vi "Main XY controller.vi"() -> ()   [LabVIEW 2015]
uses:
  <vilib>/Utility/error.llb/DialogType.ctl
  <vilib>/DAQmx/read.llb/DAQmx Read (Counter DBL 1Chan 1Samp).vi
  <vilib>/DAQmx/read.llb/DAQmx Read (Digital Bool 1Line 1Point).vi
  <vilib>/DAQmx/write.llb/DAQmx Write (Analog DBL 1Chan 1Samp).vi
  <vilib>/DAQmx/create/channels.llb/DAQmx Create Channel (DI-Digital Input).vi
  <vilib>/DAQmx/create/channels.llb/DAQmx Create Channel (CI-Count Edges).vi
  <vilib>/DAQmx/create/channels.llb/DAQmx Create Channel (AO-Voltage-Basic).vi
  <vilib>/addons/control/pid/pid.llb/PID (DBL).vi
  <vilib>/imath/engines/lvmath2/RunTimeEngine/RangeToken/NIMS_Range.vi
  <instcachedir>/0/NIMS_Range_D919CC09935940E88F755EC1C6F49AC1.lvgen/NIMS_Range_D919CC09935940E88F755EC1C6F49AC1_000.vi
  <vilib>/imathl/engines/lvmath/Functions/Error Handling/Create Error.vi
  <vilib>/imath/engines/lvmath2/RunTimeEngine/IndexRead/NIMS V(S).vi
  <instcachedir>/0/NIMS V(S)_0488751826AF41519A22953C041130DC.lvgen/NIMS V(S)_0488751826AF41519A22953C041130DC_002.vi
  <vilib>/imath/engines/lvmath2/RunTimeEngine/RowToken/NIMS_RowToken_CV_CV.vi
  <instcachedir>/0/NIMS_RowToken_CV_CV_D10E7D21517B46419B9BC15369A9C889.lvgen/NIMS_RowToken_CV_CV_D10E7D21517B46419B9BC15369A9C889_000.vi
  <vilib>/imath/engines/lvmath2/RunTimeEngine/ErrorHandling/NIMS_Create Error From Enums.vi
  <vilib>/imath/engines/lvmath2/RunTimeSupport/NIMS_Error if Not Equal.vi
  <instcachedir>/0/NIMS_Error if Not Equal_7F0D61CE56BF44979916ECA34C78675F.lvgen/NIMS_Error if Not Equal_7F0D61CE56BF44979916ECA34C78675F_001.vi
  <vilib>/imath/engines/lvmath2/RunTimeEngine/IndexRead/NIMS M(V,S).vi
  <instcachedir>/0/NIMS M(V,S)_4A7282EC9BD94252BB5D44AC841A97D6.lvgen/NIMS M(V,S)_4A7282EC9BD94252BB5D44AC841A97D6_000.vi
  <vilib>/imath/engines/lvmath2/RunTimeEngine/IndexReplace/NIMS V(V)=V.vi
  <instcachedir>/0/NIMS V(V)=V_422D7BAD0B0F4E4DA085EB3347135799.lvgen/NIMS V(V)=V_422D7BAD0B0F4E4DA085EB3347135799_000.vi
  <vilib>/imath/engines/lvmath2/RunTimeEngine/IndexRead/NIMS M($,S).vi
  <instcachedir>/0/NIMS M($,S)_3E5749BBB62E49528D4765A77F1F6D98.lvgen/NIMS M($,S)_3E5749BBB62E49528D4765A77F1F6D98_000.vi
  <vilib>/imath/engines/lvmath2/RunTimeEngine/NodeEndStatement/NIMS_NodeEndStatement_Output.vi
  <instcachedir>/0/NIMS_NodeEndStatement_Output_53EC0D466D134D7ABD903AC30B43404B.lvgen/NIMS_NodeEndStatement_Output_53EC0D466D134D7ABD903AC30B43404B_005.vi
  <vilib>/imath/engines/lvmath2/RunTimeEngine/ErrorHandling/NIMS_Finalize Error.vi
  <instcachedir>/0/NIMS_Error if Not Equal_7F0D61CE56BF44979916ECA34C78675F.lvgen/NIMS_Error if Not Equal_7F0D61CE56BF44979916ECA34C78675F_000.vi
  <instcachedir>/0/NIMS V(S)_0488751826AF41519A22953C041130DC.lvgen/NIMS V(S)_0488751826AF41519A22953C041130DC_000.vi
  <vilib>/imath/engines/lvmath2/RunTimeEngine/VariableToken/NIMS_VariableToken_CondDefined.vi
  <instcachedir>/0/NIMS_VariableToken_CondDefined_FE30D0A1BFB24F098D41DEBABFE96BE1.lvgen/NIMS_VariableToken_CondDefined_FE30D0A1BFB24F098D41DEBABFE96BE1_004.vi
  <vilib>/imath/engines/lvmath/Functions/Error Handling/MergeErrorsWrapper.vi
  <instcachedir>/0/NIMS_NodeEndStatement_Output_53EC0D466D134D7ABD903AC30B43404B.lvgen/NIMS_NodeEndStatement_Output_53EC0D466D134D7ABD903AC30B43404B_001.vi
  <vilib>/DAQmx/miscellaneous.llb/DAQmx Fill In Error Info.vi
  <vilib>/addons/control/pid/NI_PID_pid.lvlib
panel:
  out "EncoderB":dbl
  out "EncoderA":dbl
  out "StoredM2":dbl
  out "StoredM1":dbl
  out "M2":dbl format="%0.2f"
  out "M1":dbl format="%0.2f"
  out "X Response":cluster{"X Pos":dbl, "Height 2":dbl}(graph)
  in  "stop":bool
  out "X Pos":dbl
  out "Y Pos":dbl
  out "Motor 1 Voltage":dbl
  out "Motor 2 Voltage":dbl
  out "Position (mm)":cluster{"X":dbl[], "Y":dbl[]}[](graph)
  out "Left Limit LED":bool
  out "Right Limit LED":bool
  out "Bottom Limit LED":bool
  out "Top Limit LED":bool
  in  "Speed Polling Rate":dbl=0.1 caption="Time Target (s)"
  out "Motor 2 Speed":dbl(knob) scale=0.0..100.0
  out "Motor 1 Speed":dbl(knob) scale=0.0..100.0
  out "Y Response":cluster{"X Pos":dbl, "Height 2":dbl}(graph)
  out "Motor 1  Voltage":dbl(graph)
  out "Motor 2 Voltage":dbl(graph)
  in  "Motion Control":T1(tab)
  in  "Acceleration":dbl=0.1 step=0.01
  in  "DL":bool
  out "Speed":dbl
  in  "Up":bool
  in  "R":bool
  in  "L":bool
  in  "Down":bool
  in  "UR":bool
  in  "DR":bool
  in  "UL":bool
  in  "Motor Offset 1":dbl=1.0 step=0.01 format="%#_13g"
  in  "Motor Offset 2":dbl=0.96 step=0.01 format="%#_13g"
  in  "Initial Speed":dbl=5.0
  in  "Height 2":dbl
  in  "Width 2":dbl
  in  "Go to position 3":bool
  out "Drawing? 2":bool
  out "Change State Flag 2":i32
  in  "PID gains":T2={"proportional gain (Kc)"=10.0, "integral time (Ti, min)"=0.1, "derivative time (Td, min)"=0.0}
  in  "dt (s)":dbl=20.0 format="%#_13g"
  in  "Max Speed":dbl(knob) scale=0.0..10.0
  in  "Reset Button":bool caption="OK Button"
  in  "State":u32
  in  "Max Speed":dbl=7.5
  out "Drawing?":bool
  in  "Draw Circle":bool
  in  "Height":dbl=50.0
  in  "Width":dbl=20.0
  out "StartingX":dbl
  out "StartingY":dbl
  out "Y Motor Control":dbl
  out "X Motor Contorl":dbl
  in  "Allowable Error":dbl=1.0
  in  "Up Limit":tag="Dev5/port0/line0"
  in  "Bottom Limit":tag="Dev5/port0/line1"
  in  "Right Limit":tag="Dev5/port0/line2"
  in  "Left Limit":tag="Dev5/port0/line3"
  in  "Motor 1 Encoder":tag="Dev5/ctr0"
  in  "Motor 2 Encoder":tag="Dev5/ctr1"
  in  "Motor2":tag="Dev5/ao1"
  in  "Motor1":tag="Dev5/ao0"
  in  "Max Voltage":dbl
  in  "Reinitialize X & Y Pos":bool
  in  "Speed (Voltage)":dbl
  in  "Go to position 2":bool
  out "Boolean 2":bool
  in  "Desired Y":dbl
  in  "Desired X":dbl
  out "X Motor Contorl 2":dbl
  out "Y Motor Control 2":dbl
  in  "Generate coordinates":bool
  out "Drawing?":bool
  in  "draw circle":bool
  in  "Radius":dbl=50.0
  in  "Points":dbl=300.0 step=180.0
  in  "Max Speed":dbl=5.0
  in  "Allowable Error 2":dbl=0.45
  in  "Point":u32
  out "StoredM2 2":dbl
  out "StoredM1 2":dbl
  out "M2 2":dbl format="%0.2f"
  out "M1 2":dbl format="%0.2f"
  out "ypos":dbl[](array[numeric])
  out "xpos":dbl[](array[numeric])
  out "Y Motor Control 4":dbl
  out "X Motor Contorl 4":dbl
  out "Storage 2":dbl
  out "Storage":dbl
  out "Desired plot X":dbl
  out "Desired Y plot":dbl
  out "X Motor Contorl 3":dbl
  out "Y Motor Control 3":dbl
  # "Naseeb Khan - NKHA186"
  # "XY Sliderail Controller"
  # "MECHENG 312"
  # "Daniel McGinn - DMCG924"
  # "All units in mm unless otherwise specifed"
  # "Limit Switches"
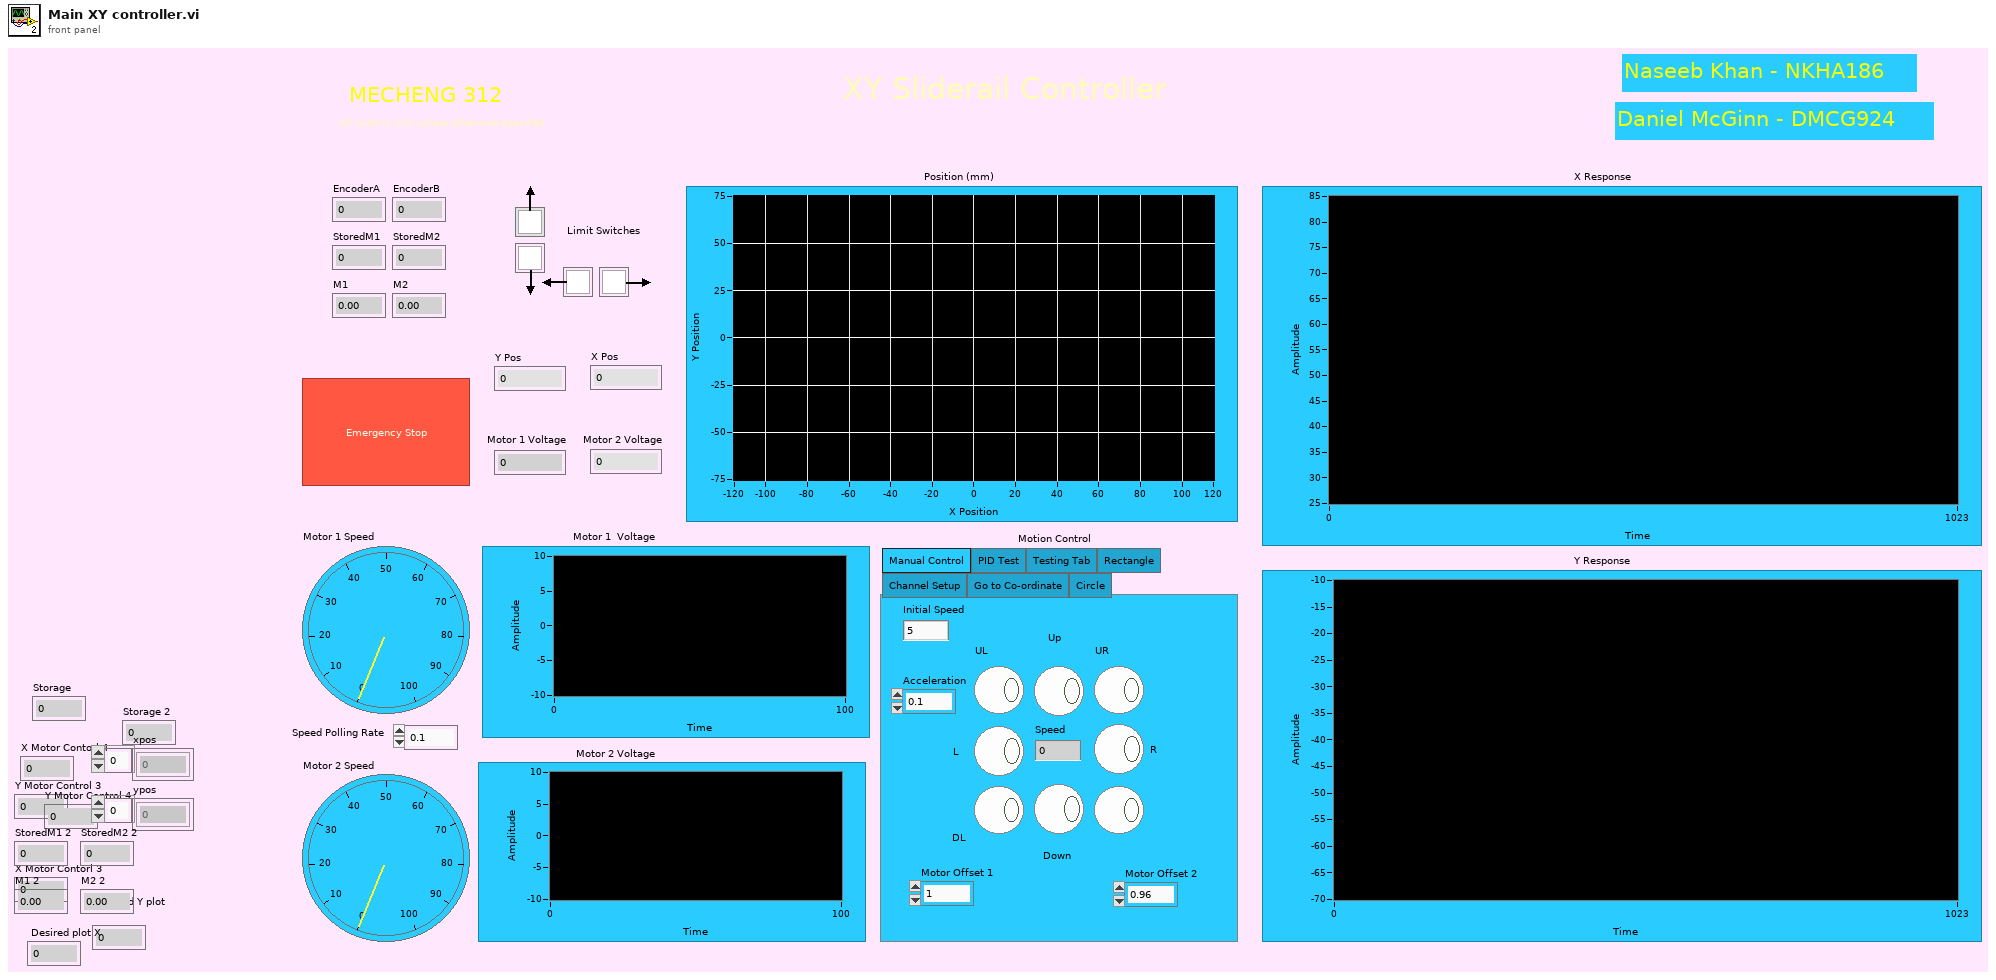
[diagram p1: front panel]
types:
  T1 = enum32{"Manual Control", "PID Test", "Testing Tab", "Rectangle", "Channel Setup", "Go to Co-ordinate", "Circle"}
  T2 = cluster{"proportional gain (Kc)":dbl, "integral time (Ti, min)":dbl, "derivative time (Td, min)":dbl}
  T3 = typedef "DialogType.ctl" = u16
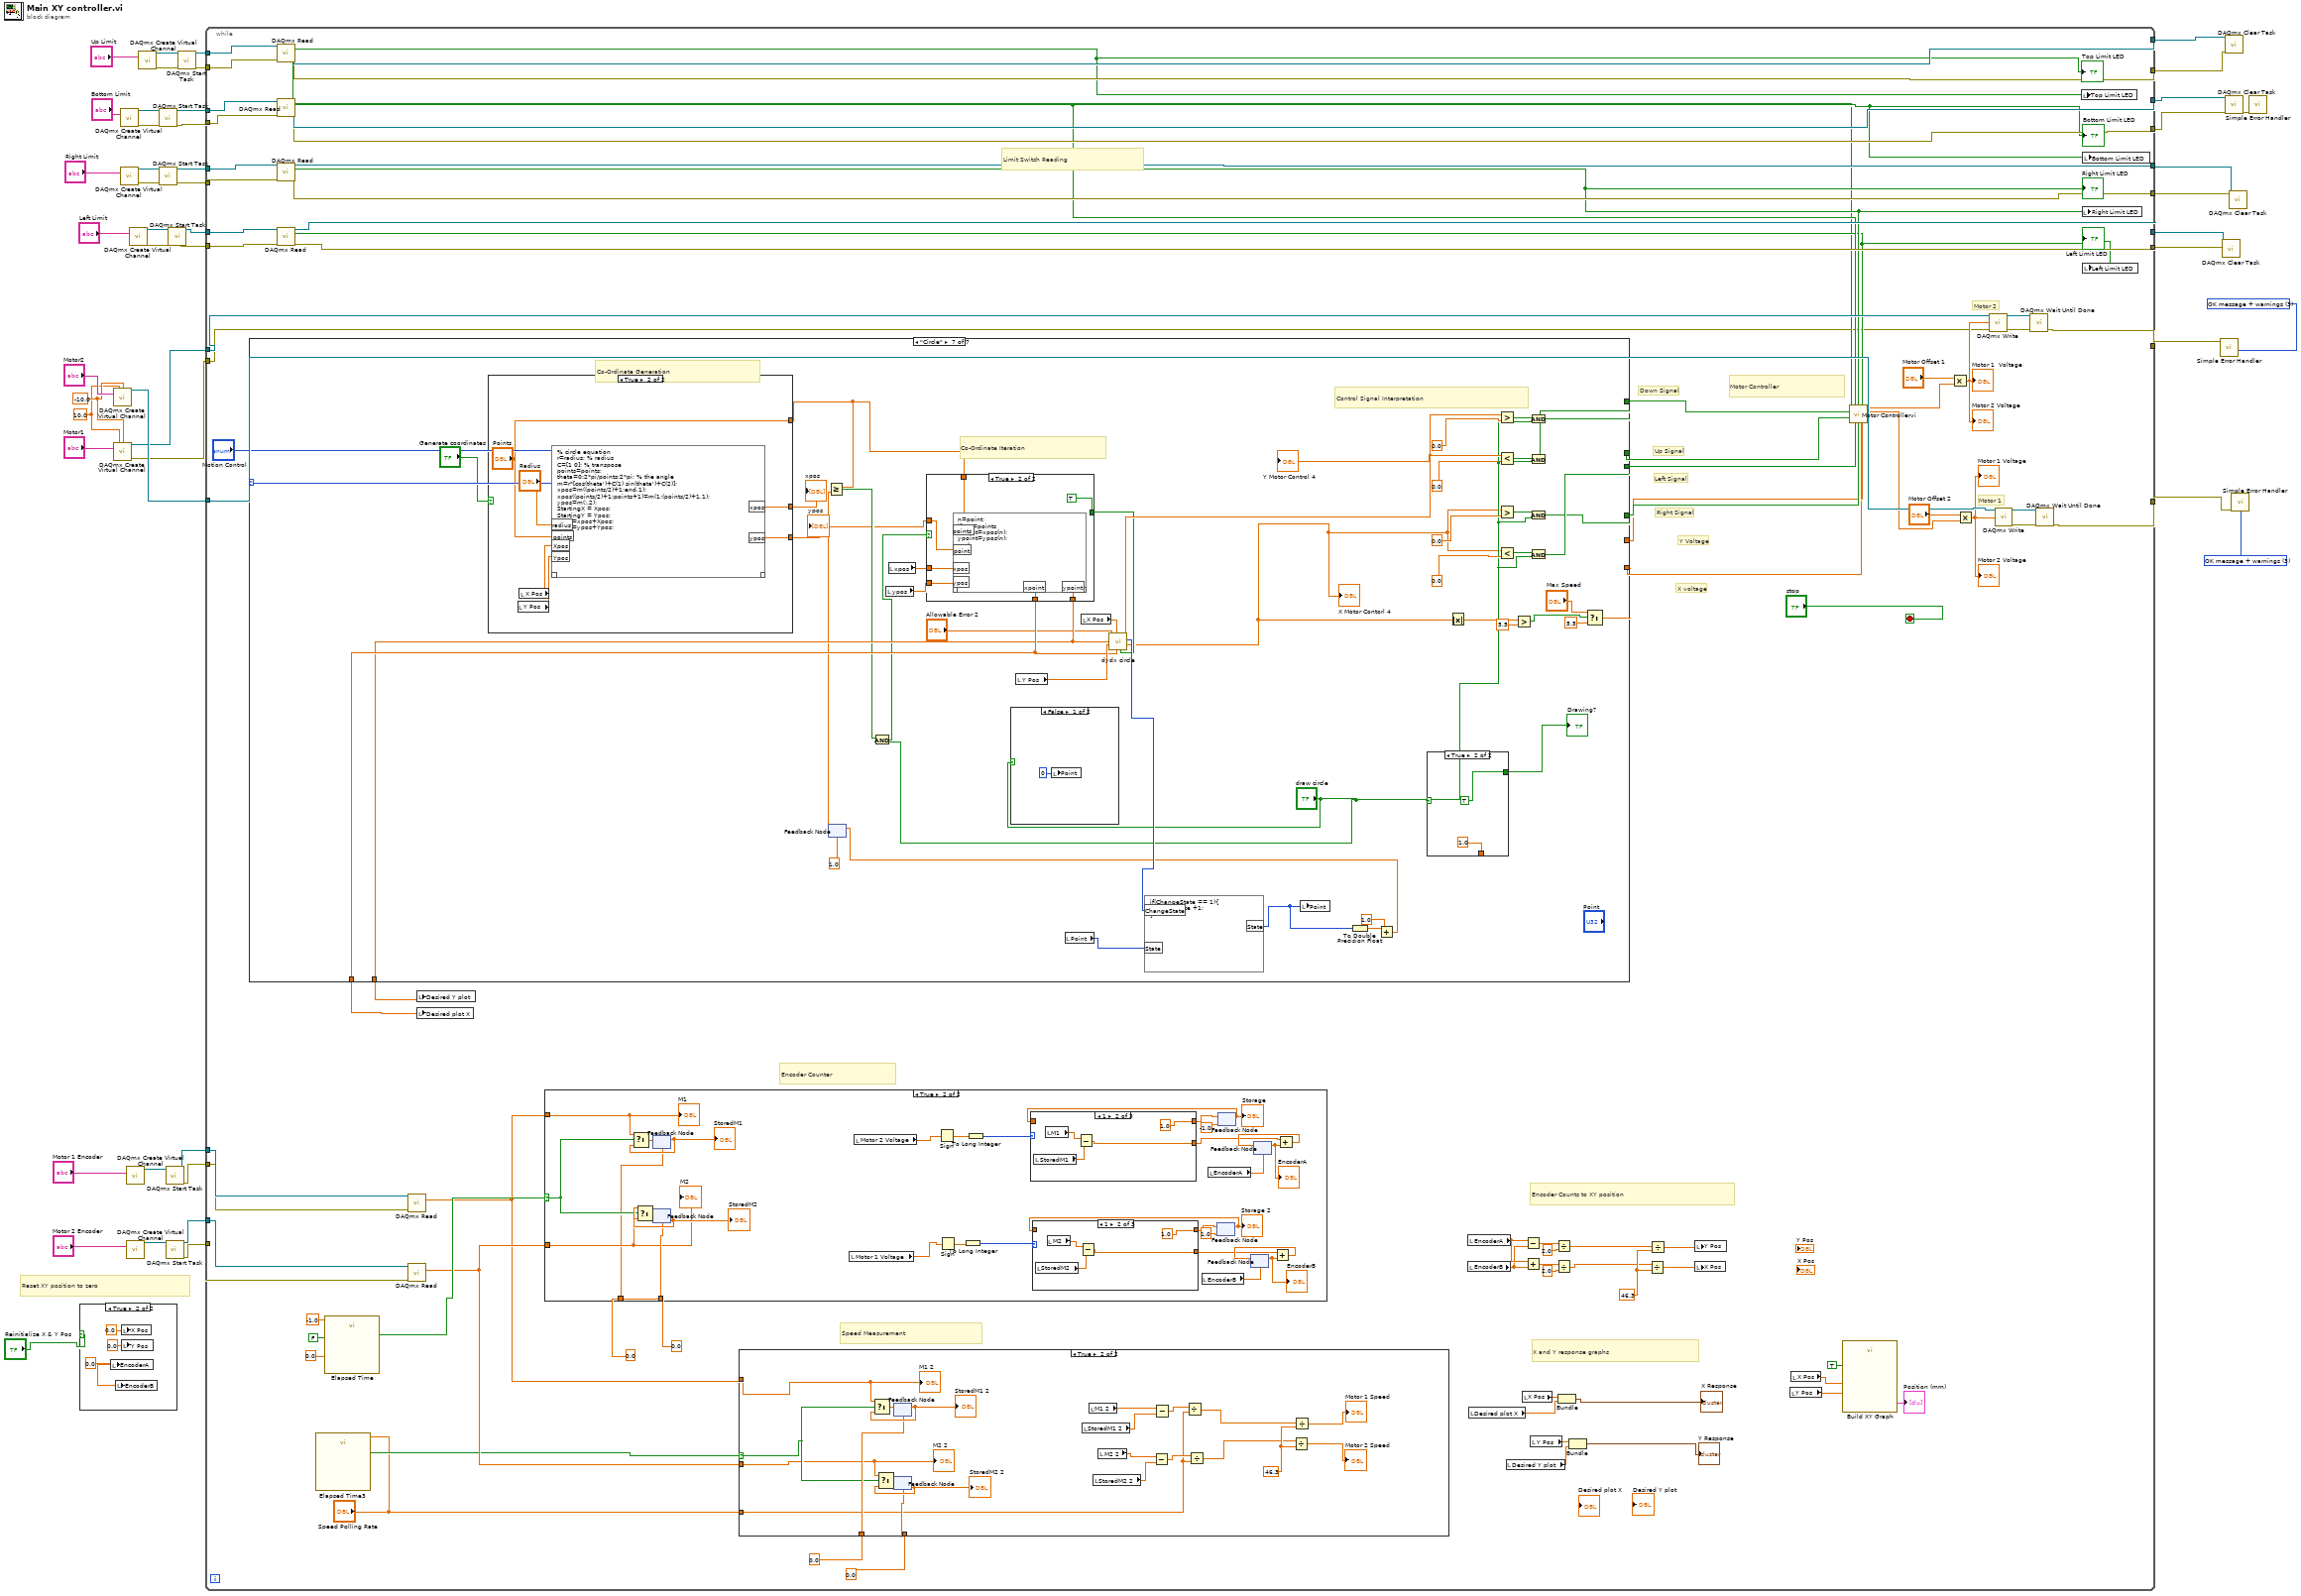
[diagram p0: block diagram]
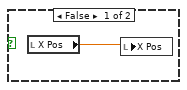
[diagram p2: hidden frame]
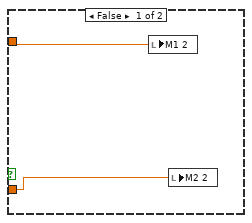
[diagram p3: hidden frame]
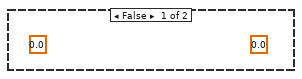
[diagram p4: hidden frame]
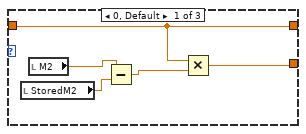
[diagram p5: hidden frame]
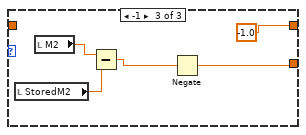
[diagram p6: hidden frame]
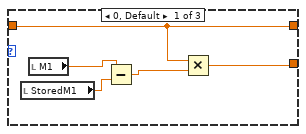
[diagram p7: hidden frame]
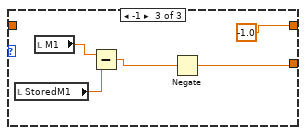
[diagram p8: hidden frame]
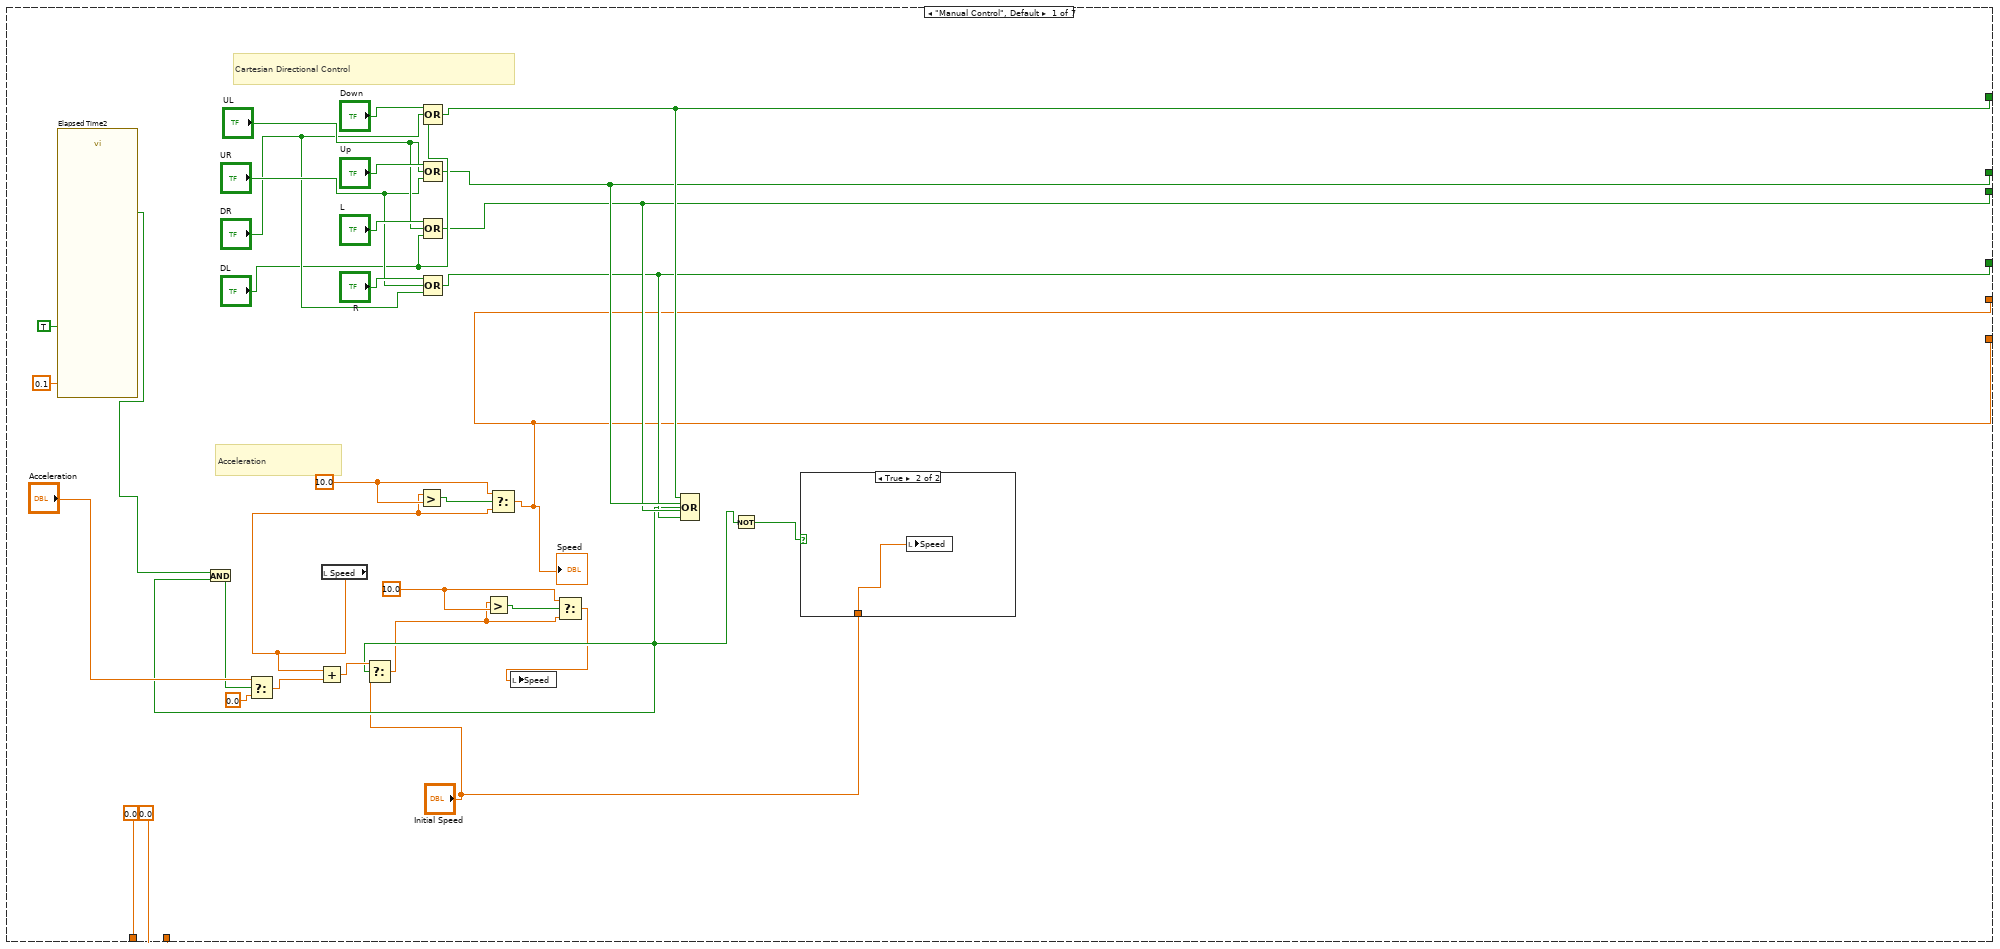
[diagram p9: hidden frame]
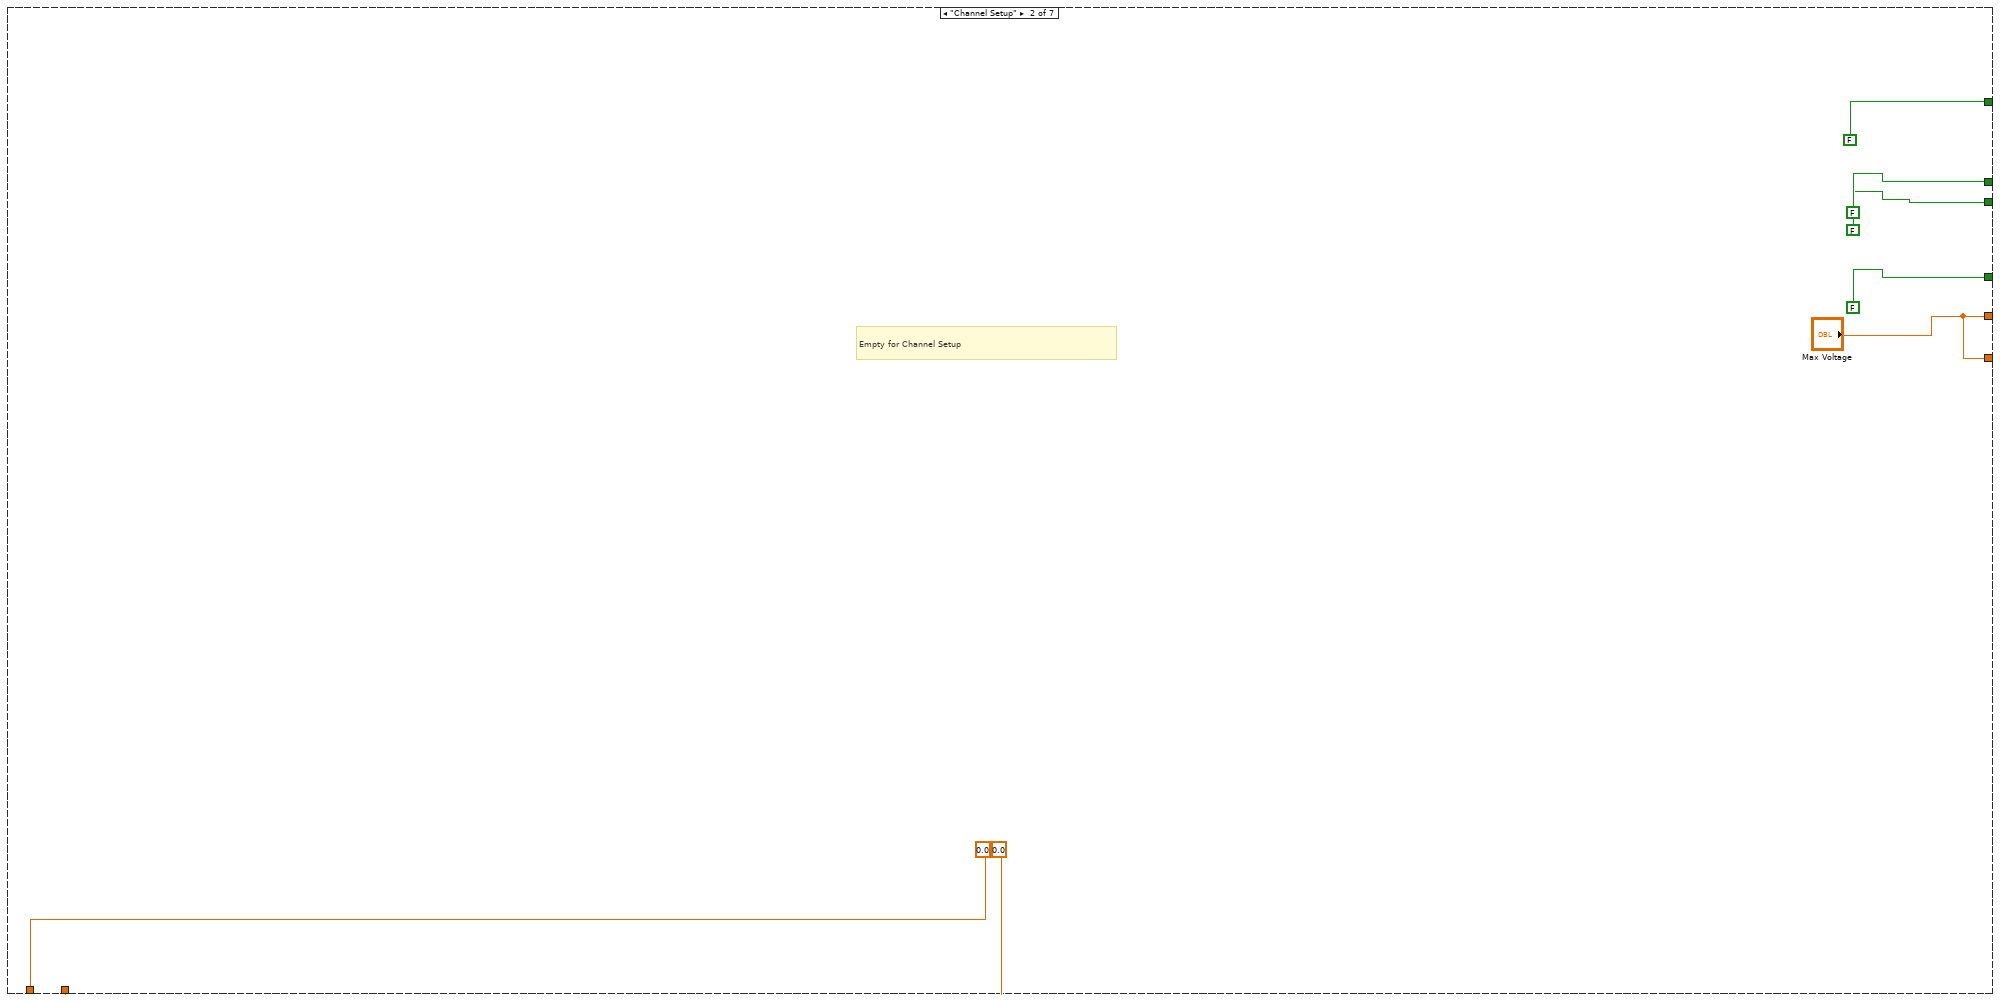
[diagram p11: hidden frame]
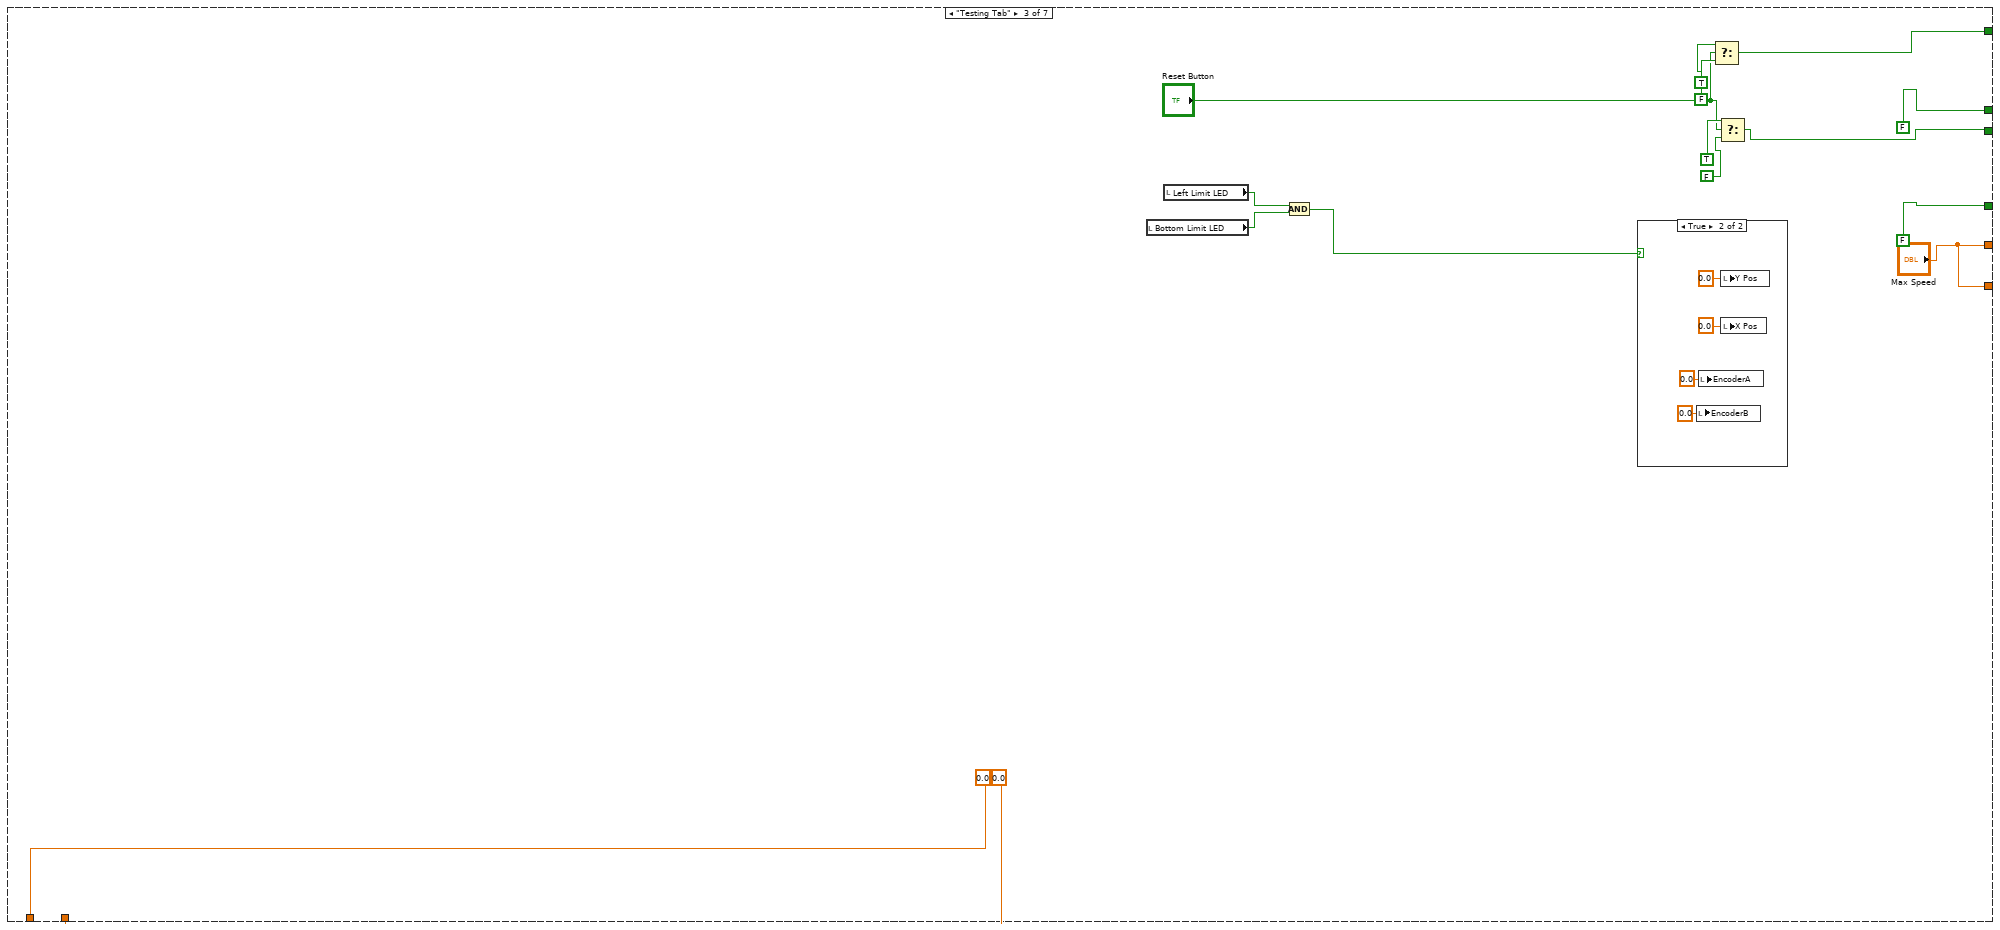
[diagram p12: hidden frame]
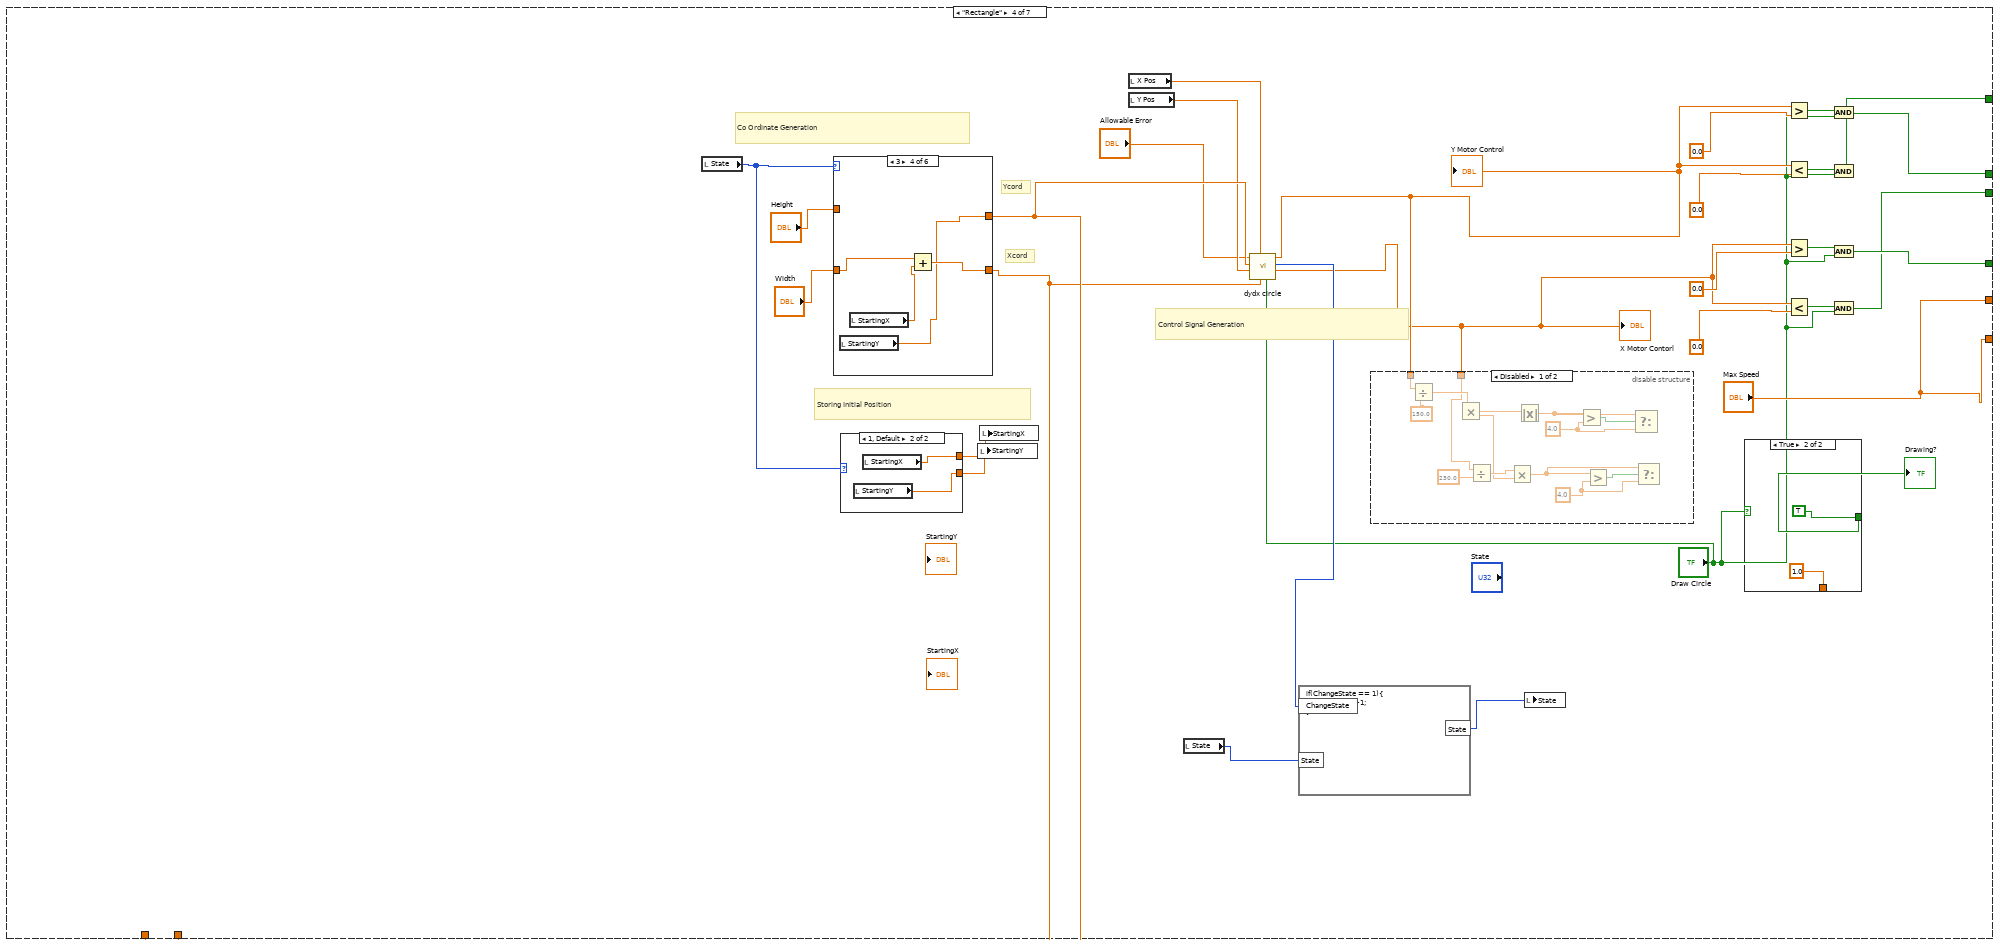
[diagram p14: hidden frame]
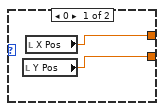
[diagram p16: hidden frame]
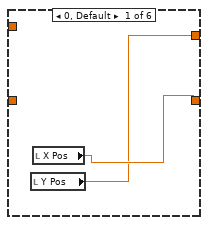
[diagram p17: hidden frame]
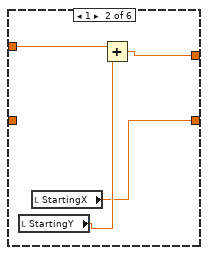
[diagram p18: hidden frame]
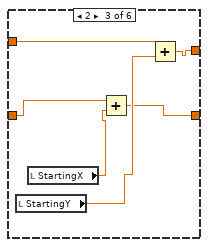
[diagram p19: hidden frame]
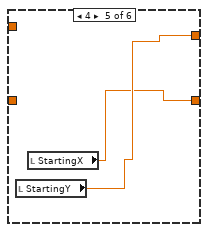
[diagram p20: hidden frame]
diagram:
  w10 = 10.0 ("Maximum Voltage")
  w11 = -10.0
  w44 = T3 3 items=["no dialog", "OK message", "continue or stop message", "OK message + warnings", "continue/stop + warnings"] ("type of dialog (OK msg:1)")
  w48 = T3 3 items=["no dialog", "OK message", "continue or stop message", "OK message + warnings", "continue/stop + warnings"] ("type of dialog (OK msg:1)")
  # "Reset XY position to zero"
  n1 = case shown="True" "Reinitialize X & Y Pos" {
    frame False {
      n2 = local read "X Pos"() -> (w50:dbl)
      n3 = local write "X Pos"(w50) -> ()
    }
    frame True {
      w51 = 0.0 ("NewEncoderPos")
      n4 = local write "EncoderA"(w51) -> ()
      n5 = local write "EncoderB"(w51) -> ()
      n6 = local write "X Pos"(0.0 ("X Pos")) -> ()
      n7 = local write "Y Pos"(0.0 ("Y Pos")) -> ()
    }
  }
  n8 = call-poly <vilib>:"DAQmx Create Virtual Channel.vi"("maximum value"=w10, "minimum value"=w11, "physical channels"="Motor2") -> ("task out"=w46:refnum<k21>)  [unwired: 11 in, 1 out]
  n9 = call-poly <vilib>:"DAQmx Create Virtual Channel.vi"("maximum value"=w10, "minimum value"=w11, "physical channels"="Motor1") -> ("task out"=w41:refnum<k21>, "error out"=w42:errorcluster)  [unwired: 11 in]
  n10 = call-poly <vilib>:"DAQmx Create Virtual Channel.vi"("lines"="Bottom Limit") -> ("task out"=w34:refnum<k21>, "error out"=w33:errorcluster)  [unwired: 13 in]
  n11 = call-poly <vilib>:"DAQmx Create Virtual Channel.vi"("lines"="Right Limit") -> ("task out"=w32:refnum<k21>, "error out"=w31:errorcluster)  [unwired: 13 in]
  n12 = call-poly <vilib>:"DAQmx Create Virtual Channel.vi"("counter"="Motor 1 Encoder") -> ("task out"=w1:refnum<k21>)  [unwired: 13 in, 1 out]
  n13 = call-poly <vilib>:"DAQmx Create Virtual Channel.vi"("counter"="Motor 2 Encoder") -> ("task out"=w7:refnum<k21>)  [unwired: 13 in, 1 out]
  n14 = call-poly <vilib>:"DAQmx Create Virtual Channel.vi"("lines"="Left Limit") -> ("task out"=w30:refnum<k21>, "error out"=w29:errorcluster)  [unwired: 13 in]
  n15 = call-poly <vilib>:"DAQmx Create Virtual Channel.vi"("lines"="Up Limit") -> ("task out"=w36:refnum<k21>, "error out"=w35:errorcluster)  [unwired: 13 in]
  n16 = call <vilib>:"DAQmx Start Task.vi"("task/channels in"=w34, "error in"=w33) -> ("task out"=w26:refnum<k21>, "error out"=w25:errorcluster)  [unwired: 12 in]
  n17 = call <vilib>:"DAQmx Start Task.vi"("task/channels in"=w32, "error in"=w31) -> ("task out"=w24:refnum<k21>, "error out"=w23:errorcluster)  [unwired: 12 in]
  n18 = call <vilib>:"DAQmx Start Task.vi"("task/channels in"=w1) -> ("task out"=w6:refnum<k21>, "error out"=w3:errorcluster)  [unwired: 13 in]
  n19 = call <vilib>:"DAQmx Start Task.vi"("task/channels in"=w7) -> ("task out"=w5:refnum<k21>, "error out"=w4:errorcluster)  [unwired: 13 in]
  n20 = call <vilib>:"DAQmx Start Task.vi"("task/channels in"=w30, "error in"=w29) -> ("task out"=w22:refnum<k21>, "error out"=w21:errorcluster)  [unwired: 12 in]
  n21 = call <vilib>:"DAQmx Start Task.vi"("task/channels in"=w36, "error in"=w35) -> ("task out"=w28:refnum<k21>, "error out"=w27:errorcluster)  [unwired: 12 in]
  n22 = while {
    tunnel: w46 -> [w133]
    tunnel: [w113] -> w45
    tunnel: [w132] -> w43
    tunnel: w42 -> [w62]
    tunnel: w41 -> [w131]
    tunnel: w28 -> [w130]
    tunnel: w27 -> [w129]
    tunnel: w26 -> [w128]
    tunnel: w25 -> [w127]
    tunnel: w24 -> [w126]
    tunnel: w23 -> [w125]
    tunnel: w22 -> [w124]
    tunnel: w21 -> [w123]
    tunnel: [w122] -> w20
    tunnel: [w121] -> w19
    tunnel: [w120] -> w18
    tunnel: [w119] -> w17
    tunnel: [w118] -> w16
    tunnel: [w117] -> w15
    tunnel: [w116] -> w14
    tunnel: [w115] -> w13
    tunnel: w6 -> [w87]
    tunnel: w5 -> [w86]
    tunnel: w4 -> [w55]
    tunnel: w3 -> [w85]
    stop <- "stop" stop-if-true
    w72 = 46.3
    # "Limit Switch Reading"
    # "Motor Controller"
    # "Speed Measurement"
    # "Encoder Counter"
    # "X and Y response graphs"
    # "Encoder Counts to XY position"
    # "Y Voltage"
    # "X voltage"
    # "Motor 1"
    # "Motor 2"
    # "Right Signal"
    # "Left Signal"
    # "Up Signal"
    # "Down Signal"
    n23 = case shown="\"Circle\"" "Motion Control" {
      tunnel: [w233 FALSE w264 w299 w377 w404 w438] -> w107
      tunnel: [w232 FALSE ("Up") FALSE ("Up") w300 w378 w405 w437] -> w106
      tunnel: [w230 FALSE ("Right\n 2") FALSE ("Right\n 2") w296 w374 w401 w435] -> w105
      tunnel: [w231 FALSE ("Left 2") w263 w295 w373 w400 w436] -> w99
      tunnel: [w220 "Max Voltage" "Max Speed" "Max Speed" w367 "Speed (Voltage)" w415] -> w97
      tunnel: [w220 "Max Voltage" "Max Speed" "Max Speed" w364 "Speed (Voltage)" w415] -> w96
      tunnel: [0.0 ("Desired Y") 0.0 ("Desired Y") 0.0 ("Desired Y") w284 "Width 2" "Desired X" w443] -> w89
      tunnel: [0.0 ("Desired X") 0.0 ("Desired X") 0.0 ("Desired X") w285 "Height 2" "Desired Y" w442] -> w88
      frame "Manual Control", Default {
        w218 = 10.0 ("y")
        w222 = 10.0 ("y")
        # "Cartesian Directional Control"
        # "Acceleration"
        n24 = call "Elapsed Time2"("Time Target (s)"=0.1, "Auto Reset"=TRUE) -> ("Time has Elapsed"=w229:bool)  [unwired: 10 in, 7 out]
        n25 = local read "Speed"() -> (w221:dbl)
        n26 = Greater?(x=w221, y=w222) -> (0:w223:bool)
        n27 = Compound Arithmetic op=OR("Down", "DR", "DL") -> (w233:bool)
        n28 = Compound Arithmetic op=OR("Up", "UL", "UR") -> (w232:bool)
        n29 = Compound Arithmetic op=OR("L", "UL", "DL") -> (w231:bool)
        n30 = Compound Arithmetic op=OR("R", "UR", "DR") -> (w230:bool)
        n31 = Select(t=w222, s=w223, f=w221) -> (s? t:f=w220:dbl)
        "Speed" <- w220
        n32 = Compound Arithmetic op=OR(w233, w232, w231, w230) -> (w225:bool)
        n33 = And(x=w229, y=w225) -> (x .and. y?=w228:bool)
        n34 = Select(t="Acceleration", s=w228, f=0.0) -> (s? t:f=w235:dbl)
        n35 = Add(x=w221, y=w235) -> (x+y=w226:dbl)
        n36 = Select(t=w226, s=w225, f="Initial Speed") -> (s? t:f=w217:dbl)
        n37 = Greater?(x=w217, y=w218) -> (0:w219:bool)
        n38 = Select(t=w218, s=w219, f=w217) -> (s? t:f=w216:dbl)
        n39 = local write "Speed"(w216) -> ()
        n40 = Not(x=w225) -> (.not. x?=w227:bool)
        n41 = case shown="True" w227 {
          tunnel: "Initial Speed" -> [_ w249]
          frame False {
          }
          frame True {
            n42 = local write "Speed"(w249) -> ()
          }
        }
      }
      frame "Channel Setup" {
        # "Empty for Channel Setup"
      }
      frame "Testing Tab" {
        n43 = local read "Bottom Limit LED"() -> (w261:bool)
        n44 = local read "Left Limit LED"() -> (w262:bool)
        n45 = And(x=w262, y=w261) -> (x .and. y?=w260:bool)
        n46 = case shown="True" w260 {
          frame False {
          }
          frame True {
            n47 = local write "EncoderB"(0.0 ("EncodB")) -> ()
            n48 = local write "EncoderA"(0.0 ("EncodA")) -> ()
            n49 = local write "Y Pos"(0.0 ("Y Pos")) -> ()
            n50 = local write "X Pos"(0.0 ("X Pos")) -> ()
          }
        }
        n51 = Select(t=TRUE, s="Reset Button", f=FALSE) -> (s? t:f=w264:bool)
        n52 = Select(t=TRUE, s="Reset Button", f=FALSE) -> (s? t:f=w263:bool)
      }
      frame "Rectangle" {
        # "Control Signal Generation"
        # "Storing Initial Position"
        # "Co Ordinate Generation"
        # "Ycord"
        # "Xcord"
        n53 = local read "State"() -> (w288:u32)
        n54 = case shown="3" w288 {
          tunnel: [w326 w327 w332 w338 w341 w343] -> w284
          tunnel: [w325 w328 w331 w337 w342 w344] -> w285
          tunnel: "Height" -> [_ w329 w336 _ _ _]
          tunnel: "Width" -> [_ _ w335 w340 _ _]
          frame 0, Default {
            n55 = local read "Y Pos"() -> (w325:dbl)
            n56 = local read "X Pos"() -> (w326:dbl)
          }
          frame 1 {
            n57 = local read "StartingY"() -> (w330:dbl)
            n58 = local read "StartingX"() -> (w327:dbl)
            n59 = Add(x=w329, y=w330) -> (x+y=w328:dbl)
          }
          frame 2 {
            n60 = local read "StartingY"() -> (w334:dbl)
            n61 = local read "StartingX"() -> (w333:dbl)
            n62 = Add(x=w335, y=w333) -> (x+y=w332:dbl)
            n63 = Add(x=w336, y=w334) -> (x+y=w331:dbl)
          }
          frame 3 {
            n64 = local read "StartingY"() -> (w337:dbl)
            n65 = local read "StartingX"() -> (w339:dbl)
            n66 = Add(x=w340, y=w339) -> (x+y=w338:dbl)
          }
          frame 4 {
            n67 = local read "StartingY"() -> (w342:dbl)
            n68 = local read "StartingX"() -> (w341:dbl)
          }
          frame 5 {
            n69 = local read "X Pos"() -> (w343:dbl)
            n70 = local read "Y Pos"() -> (w344:dbl)
            n71 = local write "State"(0) -> ()
          }
        }
        n72 = case shown="1, Default" w288 {
          tunnel: [w322 w324] -> w290
          tunnel: [w321 w323] -> w289
          frame 0 {
            n73 = local read "Y Pos"() -> (w321:dbl)
            n74 = local read "X Pos"() -> (w322:dbl)
          }
          frame 1, Default {
            n75 = local read "StartingY"() -> (w323:dbl)
            n76 = local read "StartingX"() -> (w324:dbl)
          }
        }
        n77 = local write "StartingY"(w289) -> ()
        n78 = local write "StartingX"(w290) -> ()
        n79 = local read "X Pos"() -> (w283:dbl)
        n80 = local read "Y Pos"() -> (w282:dbl)
        n81 = local read "State"() -> (w287:u32)
        n82 = call "dydx circle.vi"("count?"="Draw Circle", "Desired X in"=w284, "X Position"=w283, "Y Position"=w282, "Desired Y in"=w285, "Allowable Error 2"="Allowable Error") -> ("X Control"=w278:dbl, "ChangeState"=w280:i32, "Y Control"=w279:dbl)  [unwired: 3 in]
        "X Motor Contorl" <- w278
        "Y Motor Control" <- w279
        n83 = formula code="if(ChangeState == 1){\nState = State +1;\n}"("ChangeState"=w280, "State"=w287) -> ("State"=w286:u32)
        n84 = disable-structure shown="Disabled" {
          disable-tunnel: w279 -> [w319 _]
          disable-tunnel: w278 -> [w314 _]
          frame Disabled {
            w312 = 4.0 ("y")
            w310 = 4.0 ("y")
            n85 = Divide(x=w319, y=150.0) -> (x/y=w318:dbl)
            n86 = Multiply(x=w318) -> (y=w315:dbl, x*y=w308:dbl)
            n87 = Divide(x=w314, y=230.0) -> (x/y=w316:dbl)
            n88 = Multiply(x=w316, y=w315) -> (x*y=w306:dbl)
            n89 = Absolute Value(x=w308) -> (abs(x)=w307:dbl)
            n90 = Greater?(x=w307, y=w312) -> (0:w313:bool)
            n91 = Greater?(x=w306, y=w310) -> (0:w311:bool)
            n92 = Select(t=w307, s=w313, f=w312) -> ()  [unwired: 1 out]
            n93 = Select(t=w306, s=w311, f=w310) -> (s? t:f=w309:dbl)
          }
          frame Enabled {
          }
        }
        n94 = local write "State"(w286) -> ()
        n95 = case shown="True" "Draw Circle" {
          tunnel: [FALSE TRUE] -> w293
          tunnel: [0.0 1.0] -> _
          frame False {
          }
          frame True {
          }
        }
        "Drawing?" <- w293
        n96 = Greater?(x=w279, y=0.0) -> (0:w301:bool)
        n97 = Less?(x=w279, y=0.0) -> (x < y?=w298:bool)
        n98 = Greater?(x=w278, y=0.0) -> (0:w297:bool)
        n99 = Less?(x=w278, y=0.0) -> (x < y?=w294:bool)
        n100 = And(x=w301, y="Draw Circle") -> (x .and. y?=w300:bool)
        n101 = And(x=w298, y="Draw Circle") -> (x .and. y?=w299:bool)
        n102 = And(x=w297, y="Draw Circle") -> (x .and. y?=w296:bool)
        n103 = And(x=w294, y="Draw Circle") -> (x .and. y?=w295:bool)
      }
      frame "PID Test" {
        w365 = cluster{"output high":dbl, "output low":dbl} {"output high"=10.0, "output low"=-10.0} ("output range")
        # "Ignore"
        n104 = local read "X Pos"() -> (w363:dbl)
        n105 = local read "Y Pos"() -> (w368:dbl)
        n106 = formula code="float dY;\nfloat dX;\n\nint ChangeState = 0;\n\n dY = nextY - Yi;\n dX = nextX - Xi;\nint Xflag = 0;\nint Yflag = 0;\n\nif(( -0.5 > dY) || (dY > 0.5)){\nYcon = dY;\nYflag = 0;\n}\nelse{\nYcon = 0;\nYflag = 1;\n}\n\nif((-0.5 > dX) || (dX > 0.5)){\nXcon = dX;\nXflag = 0;\n}\nelse{\nXcon=0;\nXflag=1;\n}\n\nif((Xflag + Yflag )== 2){\nChangeState = 1;\n}"("Yi"=w368, "Xi"=w363, "nextY"="Height 2", "nextX"="Width 2") -> ("Ycon"=w359:dbl, "Xcon"=w357:dbl, "ChangeState"=→"Change State Flag 2":i32)
        n107 = call-poly <vilib>:"PID.vi"("output range"=w365, "dt (s)"="dt (s)", "PID gains"="PID gains", "process variable"=w368, "setpoint"="Height 2") -> ("output"=w353:dbl)  [unwired: 5 in, 1 out]
        "Y Motor Control 3" <- w353
        n108 = call-poly <vilib>:"PID.vi"("output range"=w365, "dt (s)"="dt (s)", "PID gains"="PID gains", "process variable"=w363, "setpoint"="Width 2") -> ("output"=w355:dbl)  [unwired: 5 in, 1 out]
        "X Motor Contorl 3" <- w355
        n109 = Equal To 0?(x=w359) -> (x = 0?=w358:bool)
        n110 = Equal To 0?(x=w357) -> (x = 0?=w356:bool)
        n111 = And(x=w358, y=w356) -> ()  [unwired: 1 out]
        n112 = case shown="True" "Go to position 3" {
          tunnel: [FALSE TRUE] -> w371
          tunnel: [0.0 1.0] -> _
          frame False {
          }
          frame True {
          }
        }
        "Drawing? 2" <- w371
        n113 = Greater?(x=w353, y=0.0) -> (0:w379:bool)
        n114 = Less?(x=w353, y=0.0) -> (x < y?=w376:bool)
        n115 = Greater?(x=w355, y=0.0) -> (0:w375:bool)
        n116 = Less?(x=w355, y=0.0) -> (x < y?=w372:bool)
        n117 = And(x=w379, y="Go to position 3") -> (x .and. y?=w378:bool)
        n118 = And(x=w376, y="Go to position 3") -> (x .and. y?=w377:bool)
        n119 = And(x=w375, y="Go to position 3") -> (x .and. y?=w374:bool)
        n120 = And(x=w372, y="Go to position 3") -> (x .and. y?=w373:bool)
        n121 = Select(t=0.0 ("f"), s=w358, f=w353) -> (s? t:f=w360:dbl)
        n122 = Select(t=0.0 ("f"), s=w356, f=w355) -> (s? t:f=w361:dbl)
        n123 = Absolute Value(x=w360) -> (abs(x)=w367:dbl)
        n124 = Absolute Value(x=w361) -> (abs(x)=w364:dbl)
      }
      frame "Go to Co-ordinate" {
        # "Basis of Rectangle and Circle Drawing"
        n125 = local read "Y Pos"() -> (w394:dbl)
        n126 = local read "X Pos"() -> (w395:dbl)
        n127 = call "dydx circle.vi"("count?"=TRUE, "Desired X in"="Desired X", "X Position"=w395, "Y Position"=w394, "Desired Y in"="Desired Y", "Allowable Error 2"=1.0) -> ("X Control"=w392:dbl, "Y Control"=w391:dbl)  [unwired: 3 in, 1 out]
        "X Motor Contorl 2" <- w392
        "Y Motor Control 2" <- w391
        n128 = case shown="True" "Go to position 2" {
          tunnel: [FALSE TRUE] -> w398
          tunnel: [0.0 1.0] -> _
          frame False {
          }
          frame True {
          }
        }
        "Boolean 2" <- w398
        n129 = Greater?(x=w391, y=0.0) -> (0:w406:bool)
        n130 = Less?(x=w391, y=0.0) -> (x < y?=w403:bool)
        n131 = Greater?(x=w392, y=0.0) -> (0:w402:bool)
        n132 = Less?(x=w392, y=0.0) -> (x < y?=w399:bool)
        n133 = And(x=w406, y="Go to position 2") -> (x .and. y?=w405:bool)
        n134 = And(x=w403, y="Go to position 2") -> (x .and. y?=w404:bool)
        n135 = And(x=w402, y="Go to position 2") -> (x .and. y?=w401:bool)
        n136 = And(x=w399, y="Go to position 2") -> (x .and. y?=w400:bool)
      }
      frame "Circle" {
        # "Control Signal Interpretation"
        # "Co-Ordinate Iteration"
        # "Co-Ordinate Generation"
        n137 = case shown="True" "Generate coordinates" {
          tunnel: [w587 "Points"] -> w423
          tunnel: [w586 w591] -> w447
          tunnel: [w585 w590] -> w446
          frame False {
            n138 = local read "Points"() -> (w587:dbl)
            n139 = local read "ypos"() -> (w585:dbl[])
            n140 = local read "xpos"() -> (w586:dbl[])
          }
          frame True {
            n141 = local read "Y Pos"() -> (w592:dbl)
            n142 = local read "X Pos"() -> (w593:dbl)
            n143 = mathscript code="% circle equation\nr=radius; % radius\nC=[1 0]; % transpose\npoints=points;\ntheta=0:2*pi/points:2*pi; % the angle\nm=r*[cos(theta')+C(1) sin(theta')+C(2)];\nxpos=m((points/2)+1:end,1); \nxpos((points/2)+1:points+1)=m(1:(points/2)+1,1);\nypos=m(:,2);\nStartingX = Xpos;\nStartingY = Ypos;\nxpos=xpos+Xpos;\nypos=ypos+Ypos;"("radius"="Radius", "points"="Points", "Xpos"=w593, "Ypos"=w592) -> ("xpos"=w591:dbl[], "ypos"=w590:dbl[])  [unwired: 1 in, 1 out]
          }
        }
        "xpos" <- w447
        "ypos" <- w446
        n144 = feedback #1(1.0) -> (w424:dbl)
        n145 = Greater Or Equal?(x=w423, y=w424) -> (x >= y?=w425:bool)
        n146 = And(x=w425, y="draw circle") -> (x .and. y?=w426:bool)
        n147 = local read "ypos"() -> (w444:dbl[])
        n148 = local read "xpos"() -> (w445:dbl[])
        n149 = case shown="True" w426 {
          tunnel: w445 -> [_ w470]
          tunnel: w444 -> [_ w469]
          tunnel: [w462 w468] -> w443
          tunnel: [w463 w467] -> w442
          tunnel: w424 -> [_ w466]
          tunnel: w423 -> [_ w465]
          tunnel: [FALSE ("count?") TRUE ("count?")] -> w427
          frame False {
            n150 = local read "X Pos"() -> (w462:dbl)
            n151 = local read "Y Pos"() -> (w463:dbl)
          }
          frame True {
            n152 = mathscript code="n=point;\nif n<=points\nxpoint=xpos(n);\nypoint=ypos(n);\nend"("point"=w466, "xpos"=w470, "ypos"=w469, "points"=w465) -> ("xpoint"=w468:dbl, "ypoint"=w467:dbl)  [unwired: 1 in, 1 out]
          }
        }
        n153 = case shown="False" "draw circle" {
          frame False {
            n154 = local write "Point"(u32 0 ("Point")) -> ()
          }
          frame True {
            n155 = local read "Point"() -> (w460:u32)
            n156 = local write "Point"(w460) -> ()
          }
        }
        n157 = local read "Y Pos"() -> (w457:dbl)
        n158 = local read "Point"() -> (w433:u32)
        n159 = local read "X Pos"() -> (w458:dbl)
        n160 = call "dydx circle.vi"("count?"=w427, "Desired X in"=w443, "X Position"=w458, "Y Position"=w457, "Desired Y in"=w442, "Allowable Error 2"="Allowable Error 2") -> ("X Control"=w417:dbl, "ChangeState"=w430:i32, "Y Control"=w448:dbl)  [unwired: 3 in]
        "X Motor Contorl 4" <- w417
        "Y Motor Control 4" <- w448
        n161 = formula code="if(ChangeState == 1){\nState = State +1;\n}"("ChangeState"=w430, "State"=w433) -> ("State"=w429:u32)
        n162 = local write "Point"(w429) -> ()
        n163 = To Double Precision Float(number=w429) -> (double precision float=w432:dbl)
        n164 = Add(x=w432, y=1.0) -> (x+y=w428:dbl)
        n165 = feedback-in #1(w428) -> ()
        n166 = case shown="True" "draw circle" {
          tunnel: [FALSE TRUE] -> w441
          tunnel: [0.0 1.0] -> _
          frame False {
          }
          frame True {
          }
        }
        "Drawing?" <- w441
        n167 = Absolute Value(x=w417) -> (abs(x)=w418:dbl)
        n168 = Greater?(x=w448, y=0.0) -> (0:w452:bool)
        n169 = Less?(x=w448, y=0.0) -> (x < y?=w451:bool)
        n170 = Greater?(x=w417, y=0.0) -> (0:w450:bool)
        n171 = Less?(x=w417, y=0.0) -> (x < y?=w449:bool)
        n172 = Greater?(x=w418, y=5.5) -> (0:w419:bool)
        n173 = And(x=w452, y="draw circle") -> (x .and. y?=w437:bool)
        n174 = And(x=w451, y="draw circle") -> (x .and. y?=w438:bool)
        n175 = And(x=w450, y="draw circle") -> (x .and. y?=w435:bool)
        n176 = And(x=w449, y="draw circle") -> (x .and. y?=w436:bool)
        n177 = Select(t="Max Speed", s=w419, f=5.5) -> (s? t:f=w415:dbl)
      }
    }
    n178 = call-poly <vilib>:"DAQmx Read.vi"("task/channels in"=w130, "error in"=w129) -> ("task out"=w116:refnum<k21>, "data"=w100:bool, "error out"=w115:errorcluster)  [unwired: 11 in]
    "Top Limit LED" <- w100
    n179 = call-poly <vilib>:"DAQmx Read.vi"("task/channels in"=w128, "error in"=w127) -> ("task out"=w118:refnum<k21>, "data"=w103:bool, "error out"=w117:errorcluster)  [unwired: 11 in]
    "Bottom Limit LED" <- w103
    n180 = call-poly <vilib>:"DAQmx Read.vi"("task/channels in"=w126, "error in"=w125) -> ("task out"=w120:refnum<k21>, "data"=w102:bool, "error out"=w119:errorcluster)  [unwired: 11 in]
    "Right Limit LED" <- w102
    n181 = call-poly <vilib>:"DAQmx Read.vi"("task/channels in"=w124, "error in"=w123) -> ("task out"=w122:refnum<k21>, "data"=w101:bool, "error out"=w121:errorcluster)  [unwired: 11 in]
    "Left Limit LED" <- w101
    n182 = call "Elapsed Time3"("Time Target (s)"="Speed Polling Rate") -> ("Time has Elapsed"=w56:bool)  [unwired: 11 in, 7 out]
    n183 = call "Elapsed Time"("Time Target (s)"=-1.0, "Auto Reset"=FALSE, "Set Start Time (s)"=0.0) -> ("Time has Elapsed"=w83:bool)  [unwired: 9 in, 7 out]
    n184 = call-poly <vilib>:"DAQmx Read.vi"("task/channels in"=w87, "error in"=w85) -> ("data"=w57:dbl)  [unwired: 11 in, 2 out]
    n185 = call-poly <vilib>:"DAQmx Read.vi"("task/channels in"=w86, "error in"=w55) -> ("data"=w58:dbl)  [unwired: 11 in, 2 out]
    n186 = local write "Desired Y plot"(w88) -> ()
    n187 = local write "Desired plot X"(w89) -> ()
    n188 = case shown="True" w83 {
      selector: w83 -> [_ w168]
      tunnel: 0.0 -> [_ w185]
      tunnel: w57 -> [_ w182]
      tunnel: w58 -> [_ w181]
      tunnel: 0.0 -> [_ w167]
      frame False {
        (unwired) 0.0
        (unwired) 0.0
      }
      frame True {
        n189 = feedback #2(w185) -> (w186:dbl)
        "StoredM2" <- w186
        n190 = Select(t=w181, s=w168, f=w186) -> (s? t:f=w187:dbl)
        n191 = feedback-in #2(w187) -> ()
        n192 = feedback #3(w167) -> (w183:dbl)
        "StoredM1" <- w183
        n193 = Select(t=w182, s=w168, f=w183) -> (s? t:f=w184:dbl)
        n194 = feedback-in #3(w184) -> ()
        n195 = local read "Motor 1 Voltage"() -> (w159:dbl)
        n196 = local read "Motor 2 Voltage"() -> (w160:dbl)
        n197 = Sign(1:w160) -> (0:w162:dbl)
        n198 = Sign(1:w159) -> (0:w164:dbl)
        n199 = To Long Integer(number=w164) -> (32bit integer=w163:i32)
        n200 = To Long Integer(number=w162) -> (32bit integer=w161:i32)
        n201 = local read "EncoderB"() -> (w166:dbl)
        n202 = local read "EncoderA"() -> (w165:dbl)
        n203 = feedback #4(1.0) -> (w173:dbl)
        "Storage 2" <- w173
        n204 = case shown="1" w163 {
          tunnel: [w189 w193 w198] -> w169
          tunnel: [w192 1.0 -1.0] -> w174
          tunnel: w173 -> [w192 _ _]
          frame 0, Default {
            n205 = local read "StoredM2"() -> (w190:dbl)
            n206 = local read "M2"() -> (w191:dbl)
            n207 = Subtract(x=w191, y=w190) -> (x-y=w188:dbl)
            n208 = Multiply(x=w192, y=w188) -> (x*y=w189:dbl)
          }
          frame 1 {
            n209 = local read "StoredM2"() -> (w195:dbl)
            n210 = local read "M2"() -> (w196:dbl)
            n211 = Subtract(x=w196, y=w195) -> (x-y=w193:dbl)
          }
          frame -1 {
            n212 = local read "StoredM2"() -> (w200:dbl)
            n213 = local read "M2"() -> (w201:dbl)
            n214 = Subtract(x=w201, y=w200) -> (x-y=w197:dbl)
            n215 = Negate(x=w197) -> (-x=w198:dbl)
          }
        }
        n216 = feedback-in #4(w174) -> ()
        n217 = feedback #5(-1.0) -> (w176:dbl)
        "Storage" <- w176
        n218 = case shown="1" w161 {
          tunnel: [w203 w207 w212] -> w178
          tunnel: [w206 1.0 -1.0] -> w177
          tunnel: w176 -> [w206 _ _]
          frame 0, Default {
            n219 = local read "StoredM1"() -> (w204:dbl)
            n220 = local read "M1"() -> (w205:dbl)
            n221 = Subtract(x=w205, y=w204) -> (x-y=w202:dbl)
            n222 = Multiply(x=w206, y=w202) -> (x*y=w203:dbl)
          }
          frame 1 {
            n223 = local read "StoredM1"() -> (w209:dbl)
            n224 = local read "M1"() -> (w210:dbl)
            n225 = Subtract(x=w210, y=w209) -> (x-y=w207:dbl)
          }
          frame -1 {
            n226 = local read "StoredM1"() -> (w214:dbl)
            n227 = local read "M1"() -> (w215:dbl)
            n228 = Subtract(x=w215, y=w214) -> (x-y=w211:dbl)
            n229 = Negate(x=w211) -> (-x=w212:dbl)
          }
        }
        n230 = feedback-in #5(w177) -> ()
        n231 = feedback #6(w166) -> (w170:dbl)
        "EncoderB" <- w170
        n232 = feedback #7(w165) -> (w179:dbl)
        "EncoderA" <- w179
        n233 = Add(x=w169, y=w170) -> (x+y=w171:dbl)
        n234 = feedback-in #6(w171) -> ()
        n235 = Add(x=w178, y=w179) -> (x+y=w180:dbl)
        n236 = feedback-in #7(w180) -> ()
        "M1" <- w182
        "M2" <- w181
      }
    }
    n237 = case shown="True" w56 {
      selector: w56 -> [_ w152]
      tunnel: 0.0 -> [_ w154]
      tunnel: 0.0 -> [_ w153]
      tunnel: w58 -> [w136 w151]
      tunnel: w57 -> [w137 w150]
      tunnel: "Speed Polling Rate" -> [_ w138]
      frame False {
        n238 = local write "M1 2"(w137) -> ()
        n239 = local write "M2 2"(w136) -> ()
      }
      frame True {
        w145 = 46.3
        n240 = feedback #8(w154) -> (w157:dbl)
        "StoredM2 2" <- w157
        n241 = Select(t=w151, s=w152, f=w157) -> (s? t:f=w158:dbl)
        n242 = feedback-in #8(w158) -> ()
        n243 = feedback #9(w153) -> (w155:dbl)
        "StoredM1 2" <- w155
        n244 = Select(t=w150, s=w152, f=w155) -> (s? t:f=w156:dbl)
        n245 = feedback-in #9(w156) -> ()
        n246 = local read "StoredM1 2"() -> (w146:dbl)
        n247 = local read "M1 2"() -> (w147:dbl)
        n248 = local read "StoredM2 2"() -> (w148:dbl)
        n249 = local read "M2 2"() -> (w149:dbl)
        n250 = Subtract(x=w149, y=w148) -> (x-y=w139:dbl)
        n251 = Subtract(x=w147, y=w146) -> (x-y=w142:dbl)
        n252 = Divide(x=w142, y=w138) -> (x/y=w141:dbl)
        n253 = Divide(x=w139, y=w138) -> (x/y=w140:dbl)
        n254 = Divide(x=w140, y=w145) -> (x/y=→"Motor 2 Speed":dbl)
        n255 = Divide(x=w141, y=w145) -> (x/y=→"Motor 1 Speed":dbl)
        "M1 2" <- w150
        "M2 2" <- w151
      }
    }
    n256 = local read "EncoderA"() -> (w76:dbl)
    n257 = local read "EncoderB"() -> (w75:dbl)
    n258 = local read "Desired plot X"() -> (w90:dbl)
    n259 = local read "Desired Y plot"() -> (w91:dbl)
    n260 = local read "X Pos"() -> (w95:dbl)
    n261 = Subtract(x=w76, y=w75) -> (x-y=w73:dbl)
    n262 = Add(x=w76, y=w75) -> (x+y=w77:dbl)
    n263 = local read "Y Pos"() -> (w93:dbl)
    n264 = Divide(x=w73, y=2.0) -> (x/y=w61:dbl)
    n265 = Divide(x=w77, y=2.0) -> (x/y=w71:dbl)
    n266 = Bundle("X Pos"=w95, "Desired plot X"=w90) -> (→"X Response":cluster{"X Pos":dbl, " Desired plot X":dbl})  [unwired: 1 in]
    n267 = Bundle("Y Pos"=w93, "Desired Y plot"=w91) -> (→"Y Response":cluster{"Y Pos ":dbl, " Desired Y plot\n":dbl})  [unwired: 1 in]
    n268 = Divide(x=w71, y=w72) -> (x/y=w70:dbl)
    n269 = Divide(x=w61, y=w72) -> (x/y=w69:dbl)
    n270 = local write "Y Pos"(w69) -> ()
    n271 = local write "X Pos"(w70) -> ()
    n272 = local read "Y Pos"() -> (w109:dbl)
    n273 = local read "X Pos"() -> (w110:dbl)
    n274 = call "Build XY Graph"("Enable"=TRUE, "Y Input"=w109, "X Input"=w110) -> ("XY Graph"=→"Position (mm)":cluster{"X":dbl[], "Y":dbl[]}[])  [unwired: 7 in, 1 out]
    n275 = call "Motor Controllervi.vi"("Up Limit"=w100, "Down Limit"=w103, "Left Limit"=w102, "Right Limit"=w101, "Down"=w107, "f"=w96, "Up"=w106, "Left"=w99, "Right\n in"=w105, "f 2"=w97) -> ("Numeric 2"=w68:dbl, "Numeric"=w64:dbl)  [unwired: 4 in]
    n276 = Multiply(x="Motor Offset 1", y=w68) -> (x*y=w67:dbl)
    "Motor 2 Voltage" <- w67
    "Motor 1  Voltage" <- w67
    n277 = Multiply(x="Motor Offset 2", y=w64) -> (x*y=w65:dbl)
    "Motor 1 Voltage" <- w65
    "Motor 2 Voltage" <- w65
    n278 = call-poly <vilib>:"DAQmx Write.vi"("task/channels in"=w131, "data"=w67, "error in"=w62) -> ("task out"=w135:refnum<k21>, "error out"=w134:errorcluster)  [unwired: 10 in, 1 out]
    n279 = call-poly <vilib>:"DAQmx Write.vi"("task/channels in"=w133, "data"=w65) -> ("task out"=w112:refnum<k21>, "error out"=w114:errorcluster)  [unwired: 11 in, 1 out]
    n280 = call <vilib>:"DAQmx Wait Until Done.vi"("task/channels in"=w135, "error in"=w134) -> ("error out"=w132:errorcluster)  [unwired: 12 in, 1 out]
    n281 = call <vilib>:"DAQmx Wait Until Done.vi"("task/channels in"=w112, "error in"=w114) -> ("error out"=w113:errorcluster)  [unwired: 12 in, 1 out]
    n282 = local write "Top Limit LED"(w100) -> ()
    n283 = local write "Right Limit LED"(w102) -> ()
    n284 = local write "Bottom Limit LED"(w103) -> ()
    n285 = local write "Left Limit LED"(w101) -> ()
  }
  n286 = call <vilib>:"Simple Error Handler.vi"("type of dialog (OK msg:1)"=w48, "error in (no error)"=w43) -> ()  [unwired: 3 in, 5 out]
  n287 = call <vilib>:"DAQmx Clear Task.vi"("task in"=w20, "error in"=w19) -> ()  [unwired: 13 in, 1 out]
  n288 = call <vilib>:"DAQmx Clear Task.vi"("task in"=w14, "error in"=w13) -> ()  [unwired: 13 in, 1 out]
  n289 = call <vilib>:"DAQmx Clear Task.vi"("task in"=w16, "error in"=w15) -> ("error out"=w12:errorcluster)  [unwired: 13 in]
  n290 = call <vilib>:"DAQmx Clear Task.vi"("task in"=w18, "error in"=w17) -> ()  [unwired: 13 in, 1 out]
  n291 = call <vilib>:"Simple Error Handler.vi"("type of dialog (OK msg:1)"=w44, "error in (no error)"=w45) -> ()  [unwired: 3 in, 5 out]
  n292 = call <vilib>:"Simple Error Handler.vi"("error in (no error)"=w12) -> ()  [unwired: 4 in, 5 out]
